vi "Send_Test_Email.vi"() -> ()   [LabVIEW 2021]
uses:
  Anemometry Sub Vis/Globals/Preference_global.vi
panel:
  out "error out":errorcluster
  in  "Extra People to Email":string[](array[string])=["p.hayden@surrey.ac.uk"]
  in  "Message":string
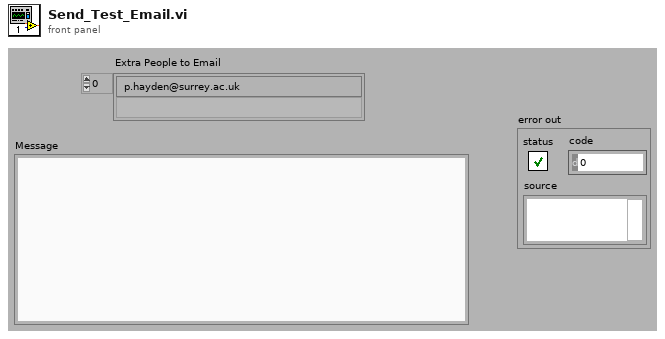
[diagram p1: front panel]
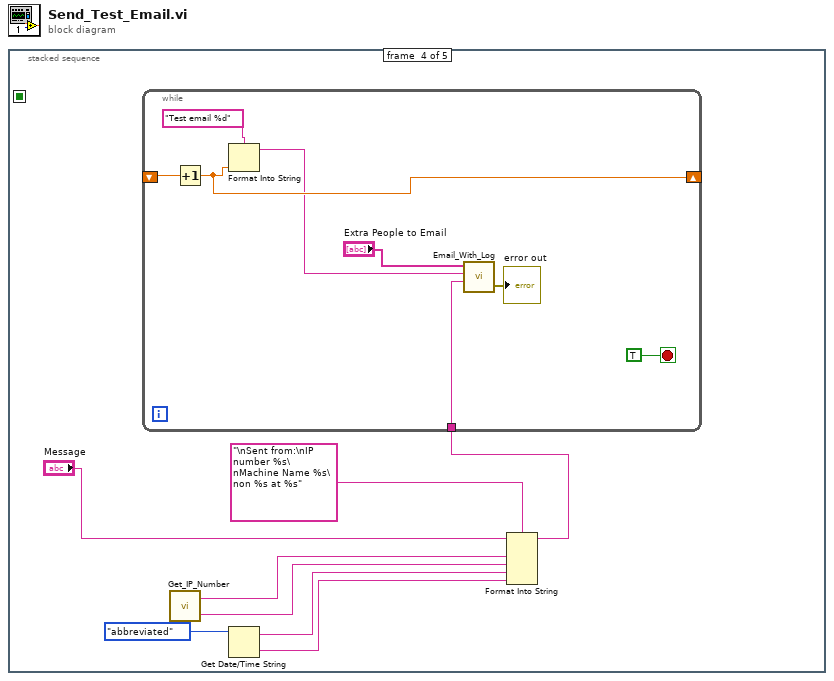
[diagram p0: block diagram]
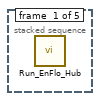
[diagram p2: hidden frame]
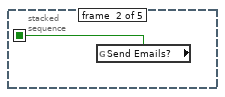
[diagram p3: hidden frame]
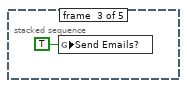
[diagram p4: hidden frame]
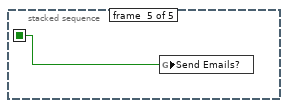
[diagram p5: hidden frame]
diagram:
  n1 = stacked-sequence {
    seq-local: [_ w1 _ _ _] -> [_ _ _ _ w19]
    frame #0 {
      n2 = call "Run_EnFlo_Hub.vi"() -> ()  [unwired: 1 in, 7 out]
    }
    frame #1 {
      n3 = global read "Preference_global.vi" "Send Emails?"() -> (w1:bool)
    }
    frame #2 {
      n4 = global write "Preference_global.vi" "Send Emails?"(TRUE ("Send Emails?")) -> ()
    }
    frame #3 {
      n5 = call "Get_IP_Number.vi"() -> ("bestAvailableName"=w8:string, "IP Number"=w9:string)
      n6 = Get Date/Time String(date format (0)=enum16{"short", "long", "abbreviated"}."abbreviated") -> (date string=w5:string, time string=w4:string)  [unwired: 1 in, 1 out]
      n7 = Format Into String(format string="\nSent from:\nIP number %s\nMachine Name %s\non %s at %s", initial string="Message", w9, w8, w5, w4) -> (resulting string=w3:string)  [unwired: 1 in, 1 out]
      n8 = while {
        shift-right: [w15] -> _
        shift-left: _ -> [w16]
        tunnel: w3 -> [w12]
        stop <- TRUE stop-if-true
        n9 = Increment(x=w16) -> (x+1=w15:dbl)
        n10 = Format Into String(format string="Test email %d" ("Error Type"), w15) -> (resulting string=w13:string)  [unwired: 2 in, 1 out]
        n11 = call "Email_With_Log.vi"("recipients"="Extra People to Email", "subject ([No Subject])"=w13, "message"=w12) -> ("error out"=→"error out":errorcluster)  [unwired: 1 in, 2 out]
      }
    }
    frame #4 {
      n12 = global write "Preference_global.vi" "Send Emails?"(w19) -> ()
    }
  }
